vi "PI Controller.vi"(8 "feedback":dbl format="%#_13g", 9 "ki":dbl format="%#_13g", 10 "kp":dbl format="%#_13g", 11 "ref":dbl format="%#_13g") -> (3 "output":dbl)   [LabVIEW 2014]
uses:
  <vilib>/Analysis/8numeric.llb/1D Numeric Integration.vi
  <vilib>/Analysis/NI_AALPro.lvlib
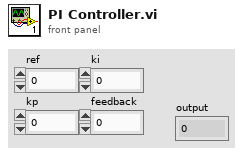
[diagram p1: front panel]
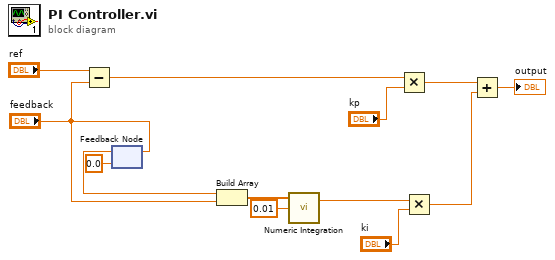
[diagram p0: block diagram]
diagram:
  n1 = Subtract(x="ref", y="feedback") -> (x-y=w9:dbl)
  n2 = feedback-in #1("feedback") -> ()
  n3 = feedback #1(0.0 ("feedback")) -> (w5:dbl)
  n4 = Build Array(w5, "feedback") -> (w4:dbl[])
  n5 = call-poly <vilib>:"Numeric Integration.vi"("dt"=0.01, "Input Array"=w4) -> ("result"=w7:dbl)  [unwired: 1 in, 1 out]
  n6 = Multiply(x=w9, y="kp") -> (x*y=w11:dbl)
  n7 = Multiply(x=w7, y="ki") -> (x*y=w2:dbl)
  n8 = Add(x=w11, y=w2) -> (x+y=→"output":dbl)
